vi "Update status display.vi"(8 "error in (no error)":errorcluster, 11 "Acquiring and Logging...":string) -> (0 "error out":errorcluster)   [LabVIEW 2020]
uses:
  Global Variables/gl_Queues.vi
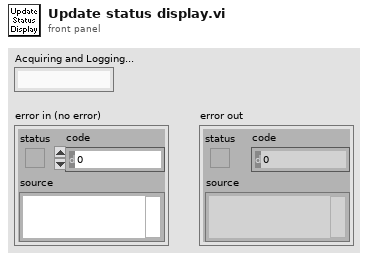
[diagram p1: front panel]
types:
  T1 = typedef "All Message Queues.ctl" = cluster{"UI queue":refnum<queue>, "Acq. queue":refnum<queue>, "Logging queue":refnum<queue>}
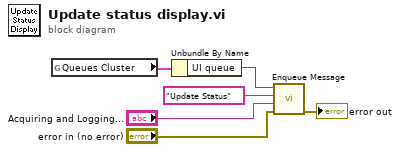
[diagram p0: block diagram]
diagram:
  n1 = global read "gl_Queues.vi" "Queues Cluster"() -> (w2:T1)
  n2 = Unbundle By Name(w2) -> ("UI queue"=w1:refnum<queue>)
  n3 = call "Enqueue Message.vi"("error in (no error)"="error in (no error)", "Message Data"="Acquiring and Logging...", "Message"="Update Status", "Queue"=w1) -> ("error out"=→"error out":errorcluster)  [unwired: 6 in, 1 out]
